vi "csv reader.vi"() -> ()   [LabVIEW 2018]
uses:
  <vilib>/Utility/file.llb/Read Delimited Spreadsheet (DBL).vi
panel:
  in  "stop 2":bool
  in  "OK Button":bool
  out "XY Graph":cluster{"Y":dbl[], "Y":dbl[]}[](graph)
  in  "stop":bool
  in  "Path":path
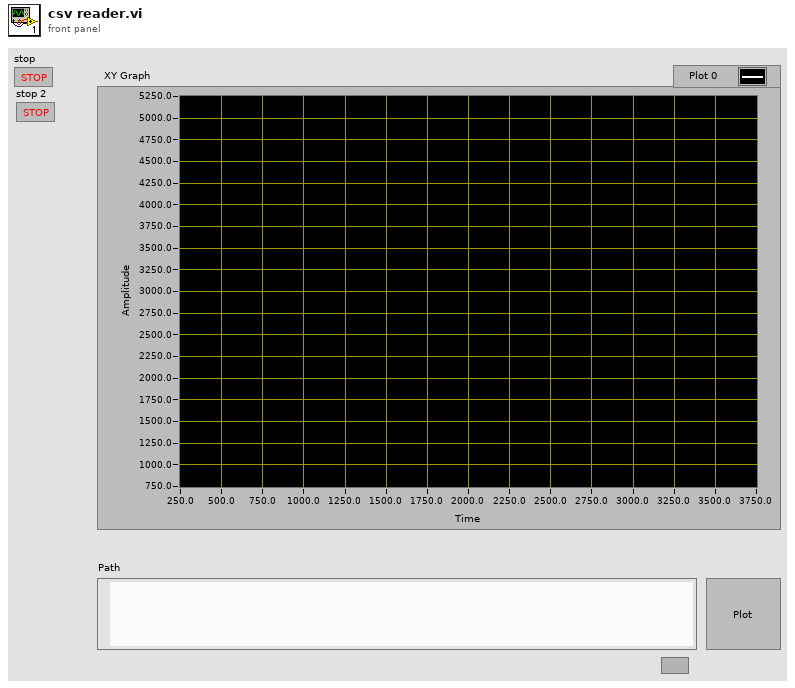
[diagram p1: front panel]
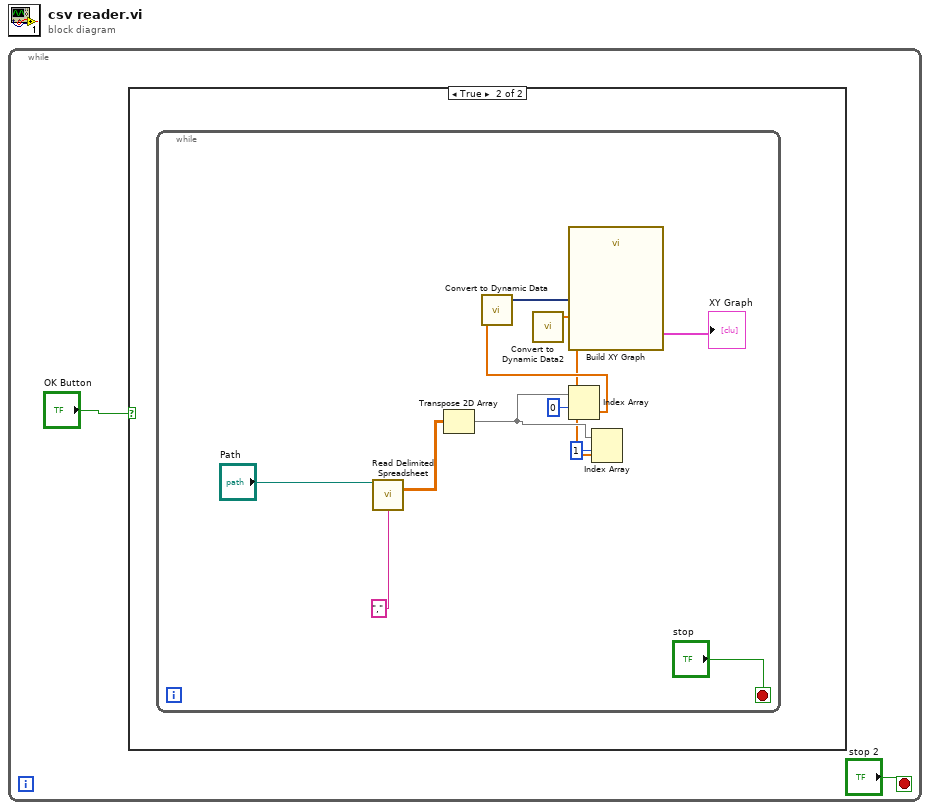
[diagram p0: block diagram]
diagram:
  n1 = while {
    stop <- "stop 2" stop-if-true
    n2 = case shown="True" "OK Button" {
      frame False {
      }
      frame True {
        n3 = while {
          stop <- "stop" stop-if-true
          n4 = call-poly <vilib>:"Read Delimited Spreadsheet.vi"("file path (dialog if empty)"="Path", "delimiter (\\t)"="," ("delimiter (\\t)")) -> ("all rows"=w10:dbl[][])  [unwired: 8 in, 5 out]
          n5 = Transpose 2D Array(2D array=w10) -> (transposed array=w6:dbl[][])
          n6 = Index Array(array=w6, index (row)=0) -> (element=w8:dbl[])  [unwired: 1 in]
          n7 = call "Convert to Dynamic Data"("Array"=w8) -> ("Dynamic Data Type"=w7:dynamicdata)  [unwired: 3 in]
          n8 = Index Array(array=w6, index (row)=1) -> (element=w4:dbl[])  [unwired: 1 in]
          n9 = call "Convert to Dynamic Data2"("Array"=w4) -> ("Dynamic Data Type"=w3:dynamicdata)  [unwired: 3 in]
          n10 = call "Build XY Graph"("Y Input"=w3, "X Input"=w7) -> ("XY Graph"=→"XY Graph":cluster{"X":dbl[], "Y":dbl[]}[])  [unwired: 8 in, 1 out]
        }
      }
    }
  }
